vi "Simple VFH Score.vi"(9 "total sample size":i32, 10 "size of best gap so far":i32, 11 "offset of best gap so far":i32) -> (3 "score":dbl)   [LabVIEW 2017, in "NI_Robotics_Simple Vector Field Histogram.lvlib"]
uses:
  <vilib>/robotics/Obstacle Avoidance/Simple Vector Field Histogram/NI_Robotics_Simple Vector Field Histogram.lvlib
  <vilib>/gmath/statdist.llb/Normal PDF.vi
  <vilib>/gmath/NI_Gmath.lvlib
panel:
  out "pdf(x)":dbl
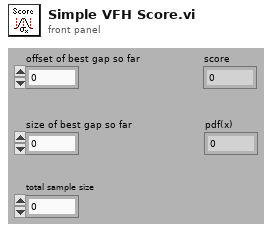
[diagram p1: front panel]
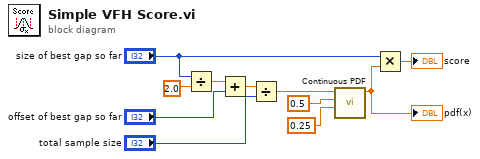
[diagram p0: block diagram]
diagram:
  n1 = Divide(x="size of best gap so far", y=2.0) -> (x/y=w7:dbl)
  n2 = Add(x=w7, y="offset of best gap so far") -> (x+y=w3:dbl)
  n3 = Divide(x=w3, y="total sample size") -> (x/y=w4:dbl)
  n4 = call-poly <vilib>:"Continuous PDF.vi"("std"=0.25, "mean"=0.5, "x"=w4) -> ("pdf(x)"=w5:dbl)  [unwired: 8 out]
  "pdf(x)" <- w5
  n5 = Multiply(x="size of best gap so far", y=w5) -> (x*y=→"score":dbl)
